vi "CorelationAnalisys.vi"() -> ()   [LabVIEW 2023]
panel:
  out "Pearson'R":dbl format="%#_2g"
  in  "Sorted":bool
  out "1D std":dbl[](array[numeric]) format="%#_4g"
  out "1D Mean":dbl[](array[numeric]) format="%#_4g"
  out "2D Mean":dbl[](array[numeric]) format="%#_4g"
  out "2D std":dbl[](array[numeric]) format="%#_4g"
  in  "Attempts":i32=8
  out "Counter":dbl
  out "x/y":dbl
  out "1D":u64[](array[numeric])
  out "2D":i32[][](array[numeric])
  out "Waveform Chart":dbl[](graph)
  out "Pearson'R":dbl[](array[numeric]) format="%#_3g"
  # "Генерира корелационните коефициенти на Пиърсън\nв зависимост от това, сортиран или не е 2D Масива."
  # ">"
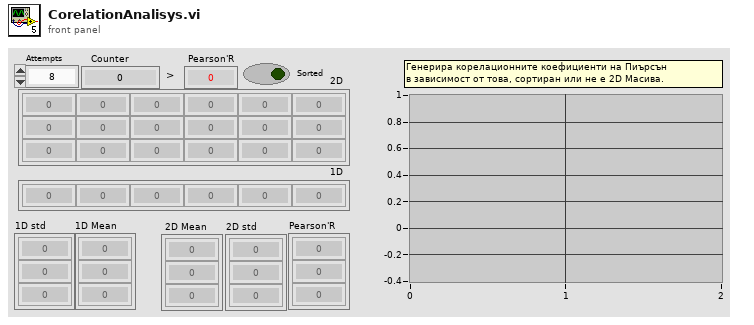
[diagram p1: front panel]
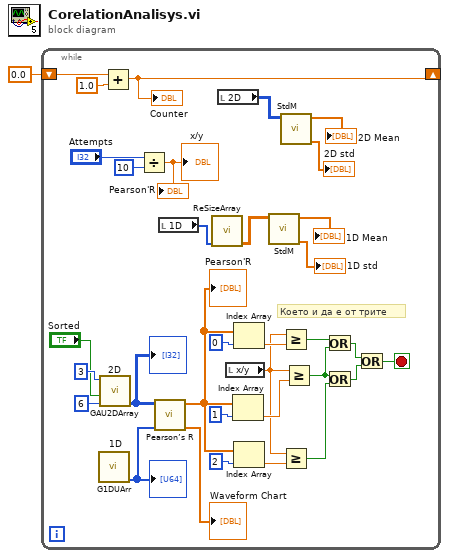
[diagram p0: block diagram]
diagram:
  n1 = while {
    shift-right: [w11] -> _
    shift-left: 0.0 -> [w10]
    stop <- w13 stop-if-true
    # "Което и да е от трите"
    n2 = call "G1DUArr.vi"() -> ("1D UArr"=w30:u64[])  [unwired: 11 in]
    "1D" <- w30
    n3 = call "GAU2DArray.vi"("Colums"=6, "Sorted"="Sorted", "Rows"=3) -> ("2D Double Array"=w31:i32[][])  [unwired: 6 in, 2 out]
    "2D" <- w31
    n4 = Add(x=w10, y=1.0) -> (x+y=w11:dbl)
    "Counter" <- w11
    n5 = Divide(x="Attempts", y=10) -> (x/y=→"x/y" →"Pearson'R":dbl)
    n6 = call "Pearson’s R.vi"("1D"=w30, "2D"=w31) -> ("kpC Chart"=→"Waveform Chart":dbl[], "kpC"=w29:dbl[])  [unwired: 8 in]
    "Pearson'R" <- w29
    n7 = local read "1D"() -> (w3:u64[])
    n8 = call "ReSizeArray.vi"("Array"=w3) -> ("1D to 2D"=w2:dbl[][])  [unwired: 9 in, 1 out]
    n9 = local read "2D"() -> (w9:i32[][])
    n10 = local read "x/y"() -> (w19:dbl)
    n11 = Index Array(array=w29, index=1) -> (element=w21:dbl)
    n12 = Index Array(array=w29, index=0) -> (element=w25:dbl)
    n13 = Index Array(array=w29, index=2) -> (element=w20:dbl)
    n14 = call "StdM.vi"("2D"=w2) -> ("My std"=→"1D std":dbl[], "Mean"=→"1D Mean":dbl[])  [unwired: 6 in, 3 out]
    n15 = call "StdM.vi"("2D"=w9) -> ("My std"=→"2D std":dbl[], "Mean"=→"2D Mean":dbl[])  [unwired: 6 in, 3 out]
    n16 = Greater Or Equal?(x=w19, y=w25) -> (x >= y?=w18:bool)
    n17 = Greater Or Equal?(x=w19, y=w20) -> (x >= y?=w17:bool)
    n18 = Greater Or Equal?(x=w19, y=w21) -> (x >= y?=w16:bool)
    n19 = Or(x=w18, y=w16) -> (x .or. y?=w14:bool)
    n20 = Or(x=w16, y=w17) -> (x .or. y?=w15:bool)
    n21 = Or(x=w14, y=w15) -> (x .or. y?=w13:bool)
  }
